vi "Close Net Use.vi"(8 "error in (no error)":errorcluster, 10 "Timeout (100s of ms)":i32=50, 11 "Net Use Drive Letter":string) -> (0 "error out":errorcluster)   [LabVIEW 2017, in "G3_Build Process File Utilities.lvlib"]
uses:
  G3_Build Process File Utilities.lvlib
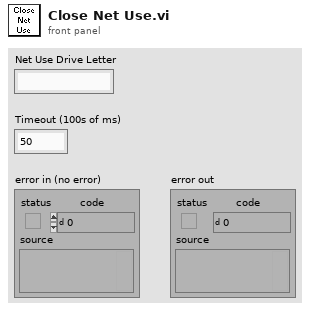
[diagram p1: front panel]
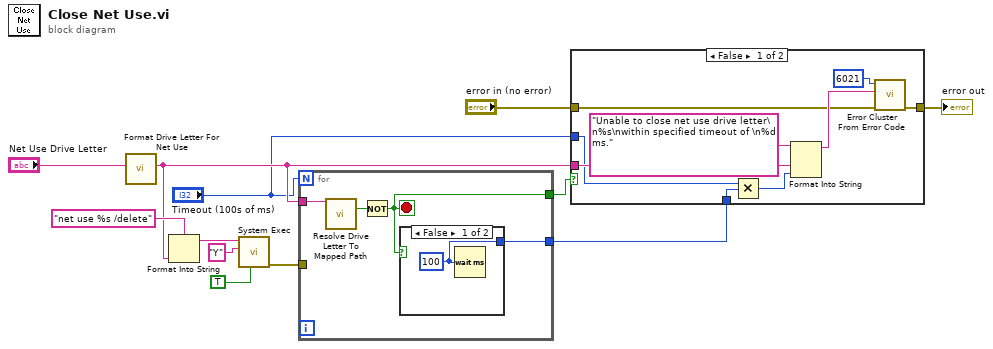
[diagram p0: block diagram]
diagram:
  n1 = call "Format Drive Letter For Net Use.vi"("Drive Letter"="Net Use Drive Letter") -> ("String"=w5:string)  [unwired: 10 in]
  n2 = Format Into String(format string="net use %s /delete", w5) -> (resulting string=w11:string)  [unwired: 2 in, 1 out]
  n3 = call <vilib>:"System Exec.vi"("run minimized? (F)"=TRUE, "standard input"="Y", "command line"=w11) -> ("error out"=w7:errorcluster)  [unwired: 5 in, 3 out]
  n4 = for {
    N: "Timeout (100s of ms)" -> [_]
    tunnel: w5 -> [w16]
    tunnel: w7 -> [_]
    tunnel: [w14] -> w6
    tunnel: [w13] -> w1
    stop <- w14 stop-if-true
    n5 = call "Resolve Drive Letter To Mapped Path.vi"("Drive Letter"=w16) -> ("Found"=w15:bool)  [unwired: 12 in, 2 out]
    n6 = Not(x=w15) -> (.not. x?=w14:bool)
    n7 = case shown="False" w14 {
      tunnel: [w17 _] -> w13
      frame False {
        w17 = u32 100 ("milliseconds to wait")
        n8 = Wait (ms)(milliseconds to wait=w17) -> ()  [unwired: 1 out]
      }
      frame True {
      }
    }
  }
  n9 = case shown="False" w6 {
    tunnel: w5 -> [w25 _]
    tunnel: [w22 w27] -> w3
    tunnel: "error in (no error)" -> [w21 w27]
    tunnel: "Timeout (100s of ms)" -> [w20 _]
    tunnel: w1 -> [w18 _]
    frame False {
      n10 = Multiply(x=w20, y=w18) -> (x*y=w19:u32)
      n11 = Format Into String(format string="Unable to close net use drive letter\n%s\nwithin specified timeout of \n%d ms.", w25, w19) -> (resulting string=w24:string)  [unwired: 2 in, 1 out]
      n12 = call <vilib>:"Error Cluster From Error Code.vi"("error in (no error)"=w21, "error message (\"\")"=w24, "error code (0)"=6021) -> ("error out"=w22:errorcluster)  [unwired: 6 in]
    }
    frame True {
    }
  }
  "error out" <- w3
